vi "AccessRequest.vi"(8 "Index":i32, 9 "KeyList":i32[](array[numeric]), 11 "InputKey":string) -> (1 "UserID":i32, 2 "IsAccess?":bool)   [LabVIEW 2016]
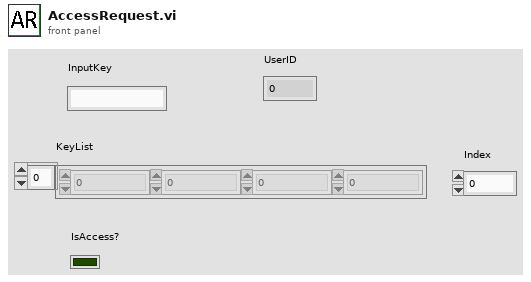
[diagram p1: front panel]
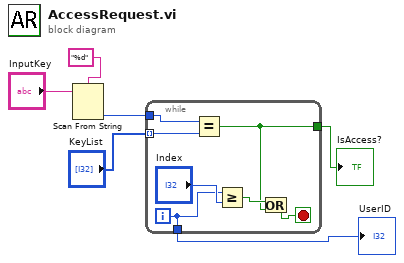
[diagram p0: block diagram]
diagram:
  n1 = Scan From String(format string="%d", input string="InputKey") -> (output 1=w3:i32)  [unwired: 3 in, 3 out]
  n2 = while {
    tunnel: "KeyList" -> [w11] mode=indexing
    tunnel: w3 -> [w12]
    tunnel: [w8] -> w2
    tunnel: [w7] -> w1
    i -> [w7]
    stop <- w9 stop-if-true
    n3 = Equal?(x=w12, y=w11) -> (x = y?=w8:bool)
    n4 = Greater Or Equal?(x=w7, y="Index") -> (x >= y?=w10:bool)
    n5 = Or(x=w10, y=w8) -> (x .or. y?=w9:bool)
  }
  "IsAccess?" <- w2
  "UserID" <- w1
